vi "Handle Command.vi"(8 "error in (no error)":errorcluster, 10 "CMD in":refnum<class "Change PMT Gain CMD.lvclass">, 11 "Object In":refnum<class>) -> (0 "error out":errorcluster, 1 "Command Successful?":bool, 2 "CMD out":refnum<class "Change PMT Gain CMD.lvclass">, 3 "Object Out":refnum<class>)   [LabVIEW 2014, in "eCRDS Library.lvlib" / "Change PMT Gain CMD.lvclass"]
doc: "This VI will contain the code used to actually execute the request. If the request is successful, this will be indicated by the boolean output <b>Command Successful?</b>. The boolean output can then be used by the <b>Command Reply</b> which sends a reply if the reply queue is valid."
uses:
  Change PMT Gain CMD.lvclass
  reusable/Instrument/Instrument.lvclass
  reusable/Instrument/Instrument.lvclass/Instrument.ctl
  Change PMT Gain CMD.lvclass/Change PMT Gain CMD.ctl
  reusable/Instrument/Read Log Session.vi
  <vilib>/DAQmx/write.llb/DAQmx Write (Analog 1D DBL NChan 1Samp).vi
  <userlib>/_Session Fwk/Session - Root.lvclass
  reusable/Session APIs/Session Log/System Log.lvclass
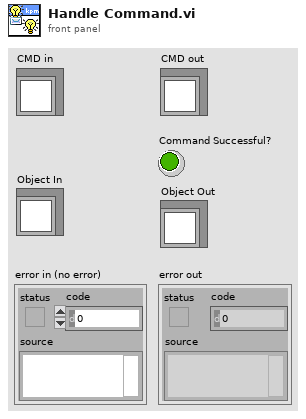
[diagram p1: front panel]
types:
  T1 = typedef "Session - Root.lvclass/Session Handle.ctl" = refnum<data-value>
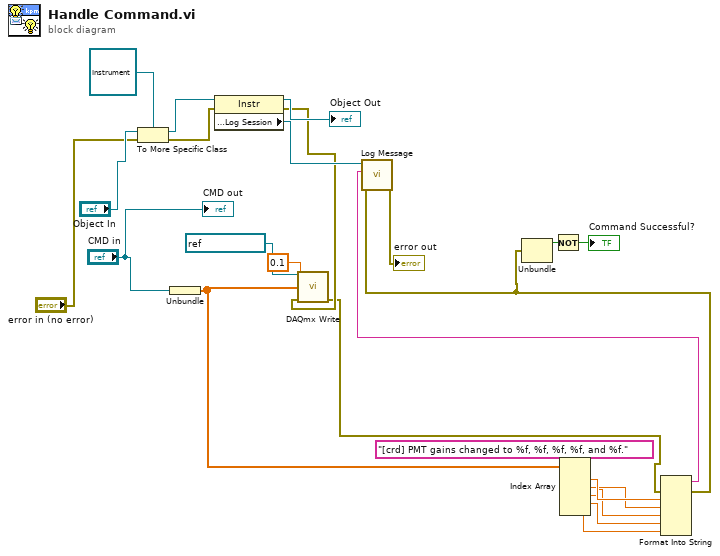
[diagram p0: block diagram]
diagram:
  (unwired) "[crd] PMT gains changed to %f, %f, %f, %f, and %f." ("format string")
  n1 = To More Specific Class(target class=refnum<class "Instrument.lvclass"> refnum ("Instr"), reference="Object In", error in="error in (no error)") -> (specific class reference=w21:refnum<class "Instrument.lvclass">, error out=w6:errorcluster)
  n2 = Unbundle("CMD in") -> (w2:dbl[])
  n3 = property class="Instr"(reference=w21, error in=w6) -> (reference out=→"Object Out":refnum<class "Instrument.lvclass">, error out=w3:errorcluster, "Accessors:Log Session"=w19:T1)
  n4 = call-poly <vilib>:"DAQmx Write.vi"("task/channels in"=refnum<k21> "PMT Gain", "data"=w2, "timeout"=0.1, "error in"=w3) -> ("error out"=w1:errorcluster)  [unwired: 9 in, 2 out]
  n5 = Index Array(array=w2) -> (element #1=w17:dbl, element #2=w16:dbl, element #3=w15:dbl, element #4=w14:dbl, element #5=w13:dbl)  [unwired: 5 in]
  n6 = Format Into String(error in=w1, w17, w16, w15, w14, w13) -> (resulting string=w11:string, error out=w10:errorcluster)  [unwired: 2 in]
  n7 = call "Log Message.vi"("error in"=w10, "MSG In"=w11, "session in"=w19) -> ("error out"=→"error out":errorcluster)  [unwired: 7 in, 1 out]
  n8 = Unbundle(w10) -> ("status"=w9:bool)  [unwired: 2 out]
  n9 = Not(x=w9) -> (.not. x?=→"Command Successful?":bool)
  "CMD out" <- "CMD in"
